vi "Main.vi"() -> ()   [LabVIEW 2016]
uses:
  State.ctl
  <vilib>/DAQmx/write.llb/DAQmx Write (Digital Bool 1Line 1Point).vi
  <vilib>/DAQmx/read.llb/DAQmx Read (Digital Bool 1Line 1Point).vi
  <vilib>/DAQmx/create/channels.llb/DAQmx Create Channel (DI-Digital Input).vi
  <vilib>/DAQmx/create/channels.llb/DAQmx Create Channel (DO-Digital Output).vi
  <vilib>/DAQmx/miscellaneous.llb/DAQmx Fill In Error Info.vi
panel:
  out "Path":path
  out "Pegs Left":dbl
  out "Rings Left":dbl
  in  "Reject Control":bool
  in  "Hopper Control":bool
  in  "Sort  Control":bool
  out "Hopper  Actuator":bool
  out "Reject Solenoid":bool
  out "Sort Solenoid":bool
  in  "Feeder Control":bool
  out "No. Rings Rej":dbl
  out "No. Pegs Rej":dbl
  in  "Belt Control":bool
  out "Rings":dbl
  out "Pegs":dbl
  out "No. Rejected":dbl
  out "No.  Assembled":dbl
  out "Ring Queue":dbl
  out "Reject Solenoid Return":bool
  out "Reject Area Detect":bool
  out "Sensing Area Detect":bool
  out "Sensing Ring Detect":bool
  out "Sensing Peg Detect":bool
  out "Hopper Full":bool
  out "Sort Solenoid Return":bool
  out "Feeder Light":bool
  out "Belt Light":bool
  out "Sort Metal Peg Detect":bool
  out "State":T1
  out "Sorting Area Detect":bool
  out "Off Light":bool
  out "Pause light":bool
  out "On light":bool
  in  "Reset Button":bool
  in  "Abort & Exit Button":bool
  in  "Stop Button":bool
  in  "Pause Button":bool
  in  "Play Button":bool
  out "Peg Flag":bool
  out "Rejection Control":i8
  out "Assembly Flag":bool
  out "Program Control":bool
  # "System Data"
  # "Sensors Panel"
  # "STATUS"
  # "STOP"
  # "READY"
  # "GO!"
  # "ICT3 Controller \nMSE 310 Course Project\nNavjot Singh - 301277656\nNeeraj Bansal - 301323495\nElvis Eshikena - 301302117\nSep - Nov 2018"
  # "Actuators Panel"
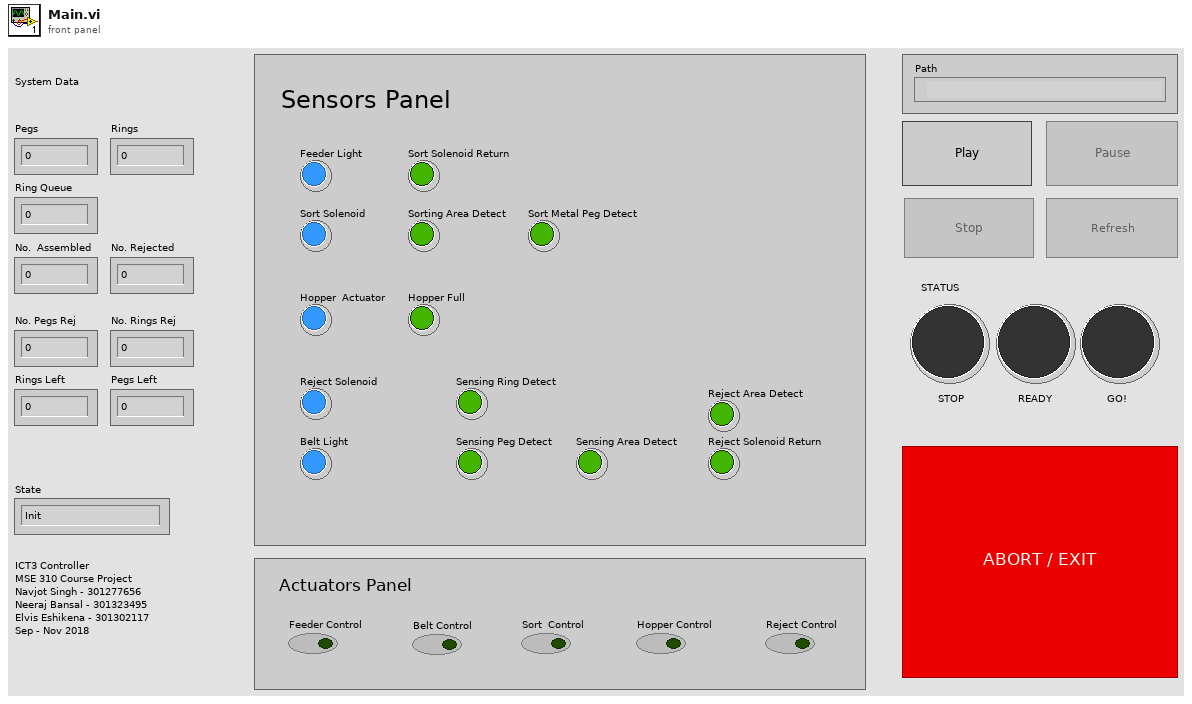
[diagram p1: front panel]
types:
  T1 = typedef "State.ctl" = enum16{"Init", "Idle", "Play", "Pause", "Reset", "Stop", "Stop Program"}
  T2 = enum8{"Enabled", "Disabled", "Disabled and Grayed Out"}
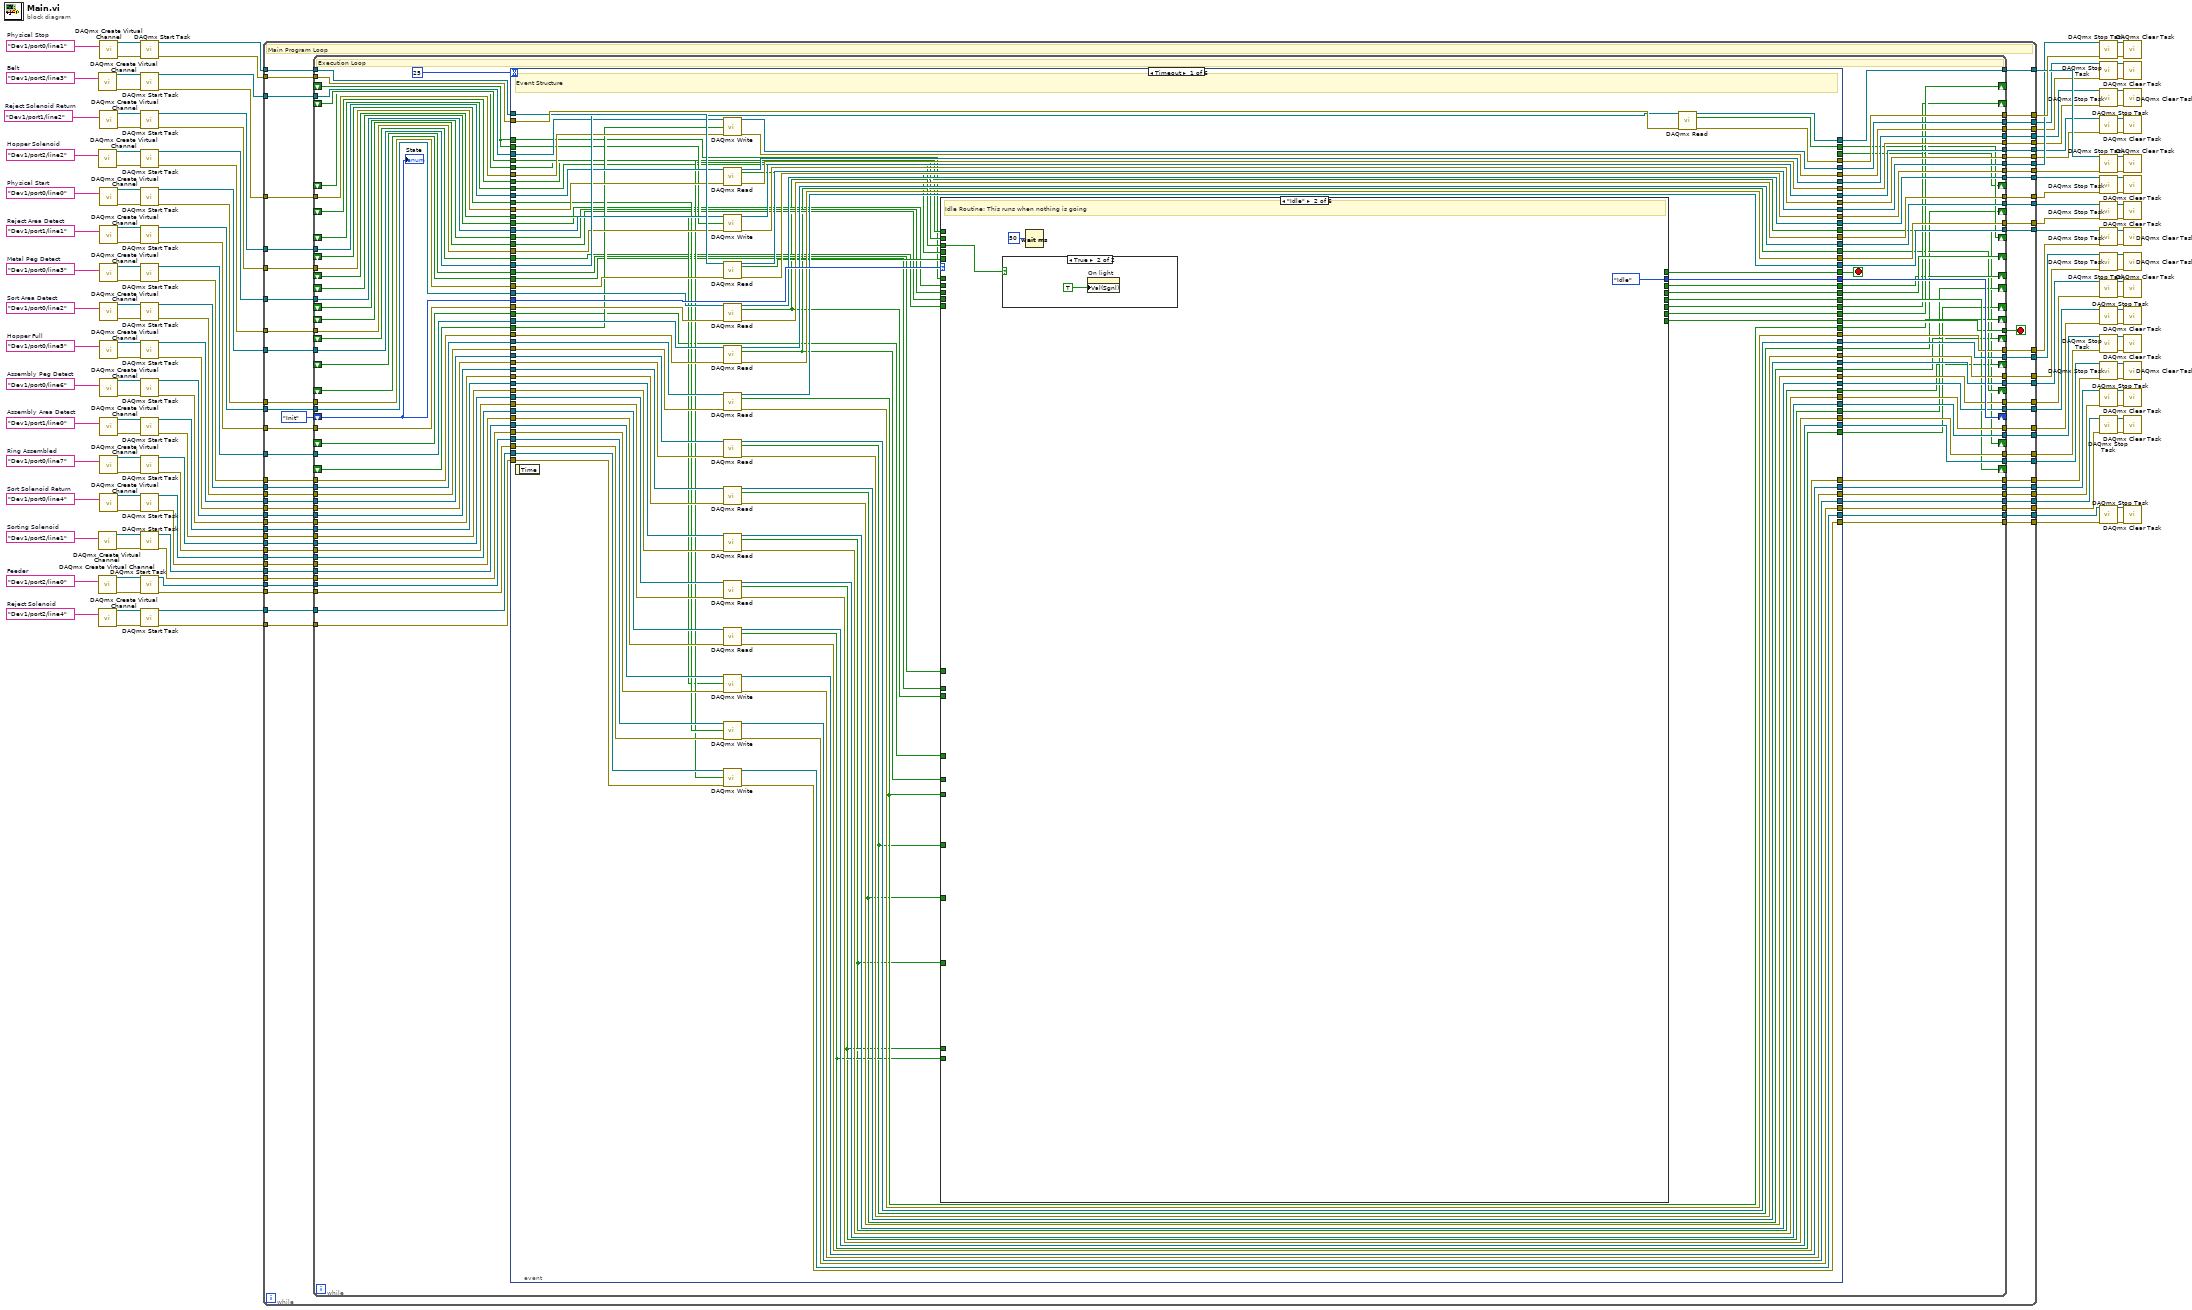
[diagram p0: block diagram]
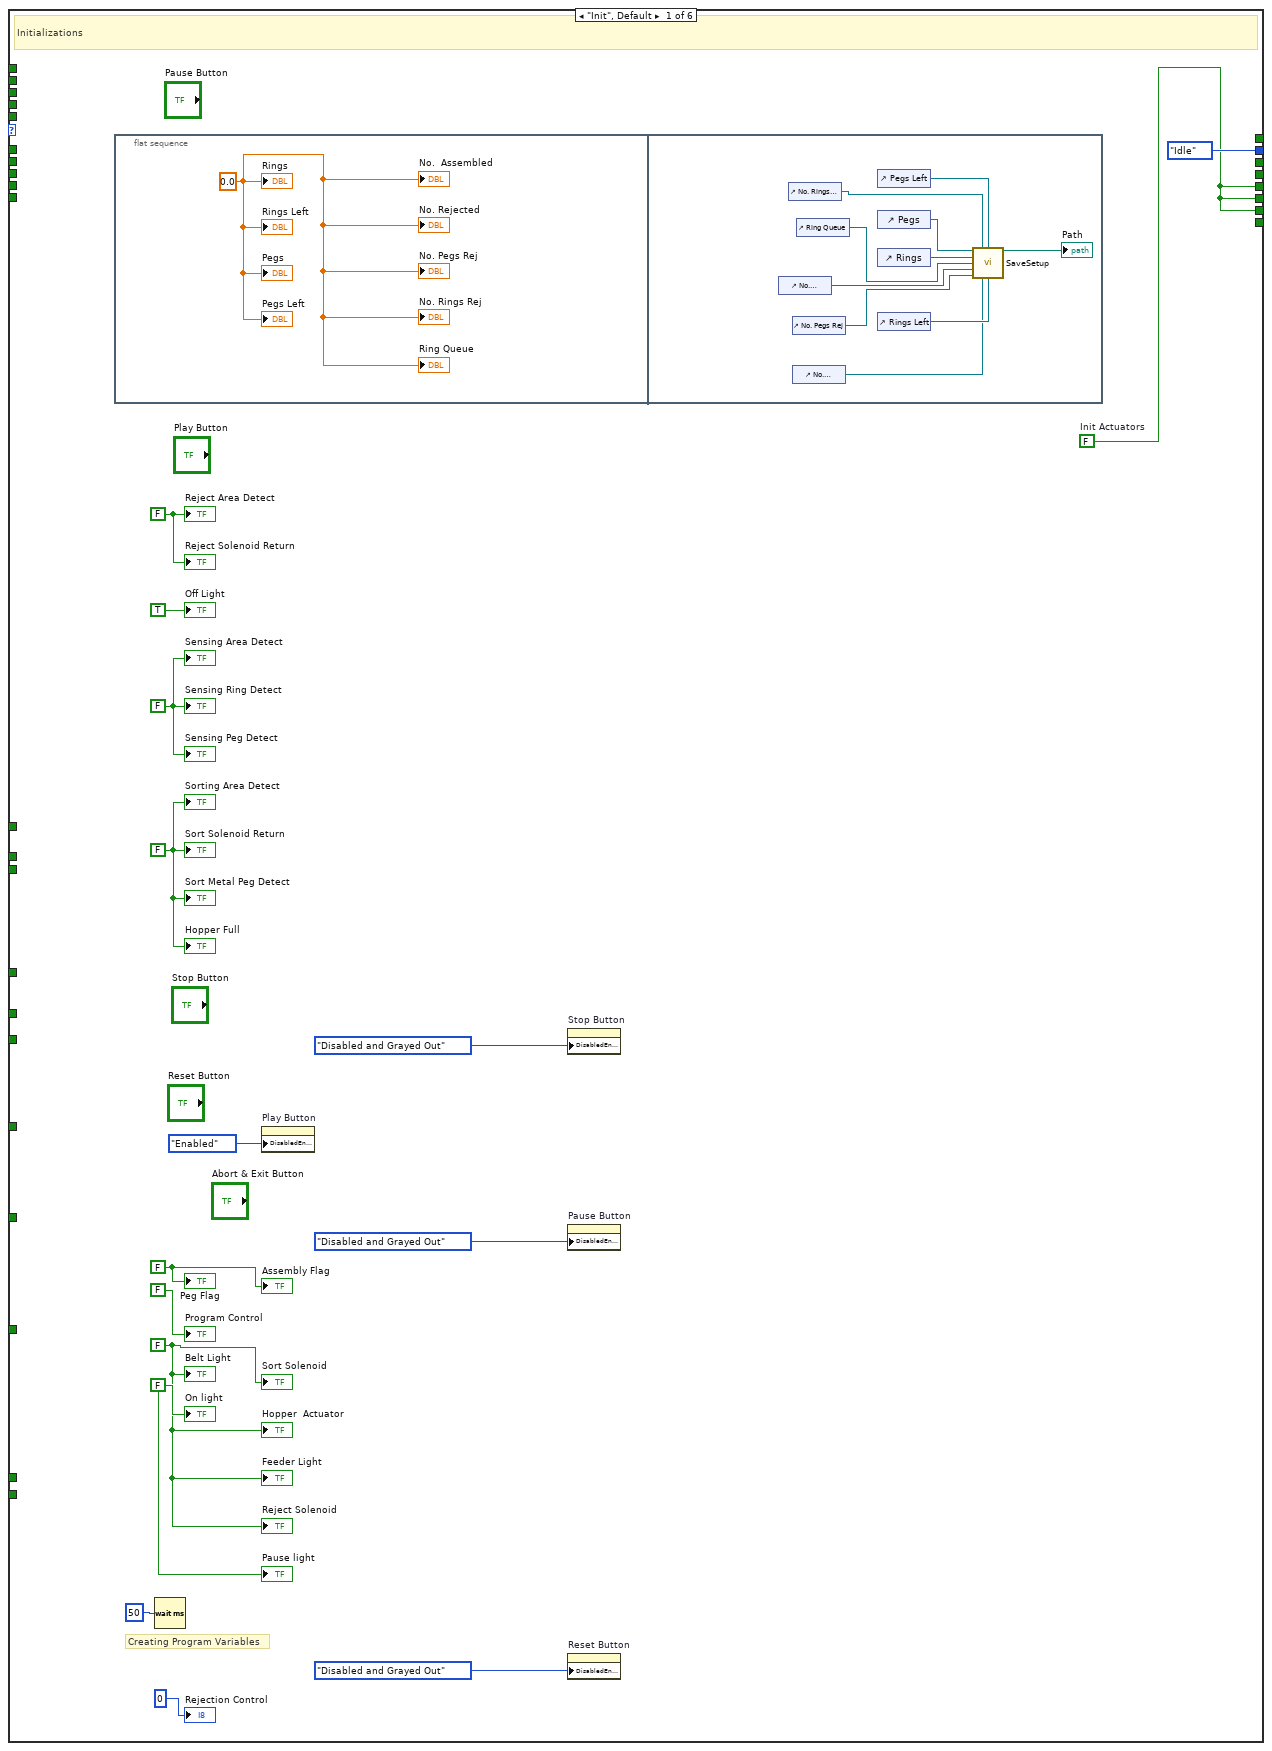
[diagram p2: hidden frame]
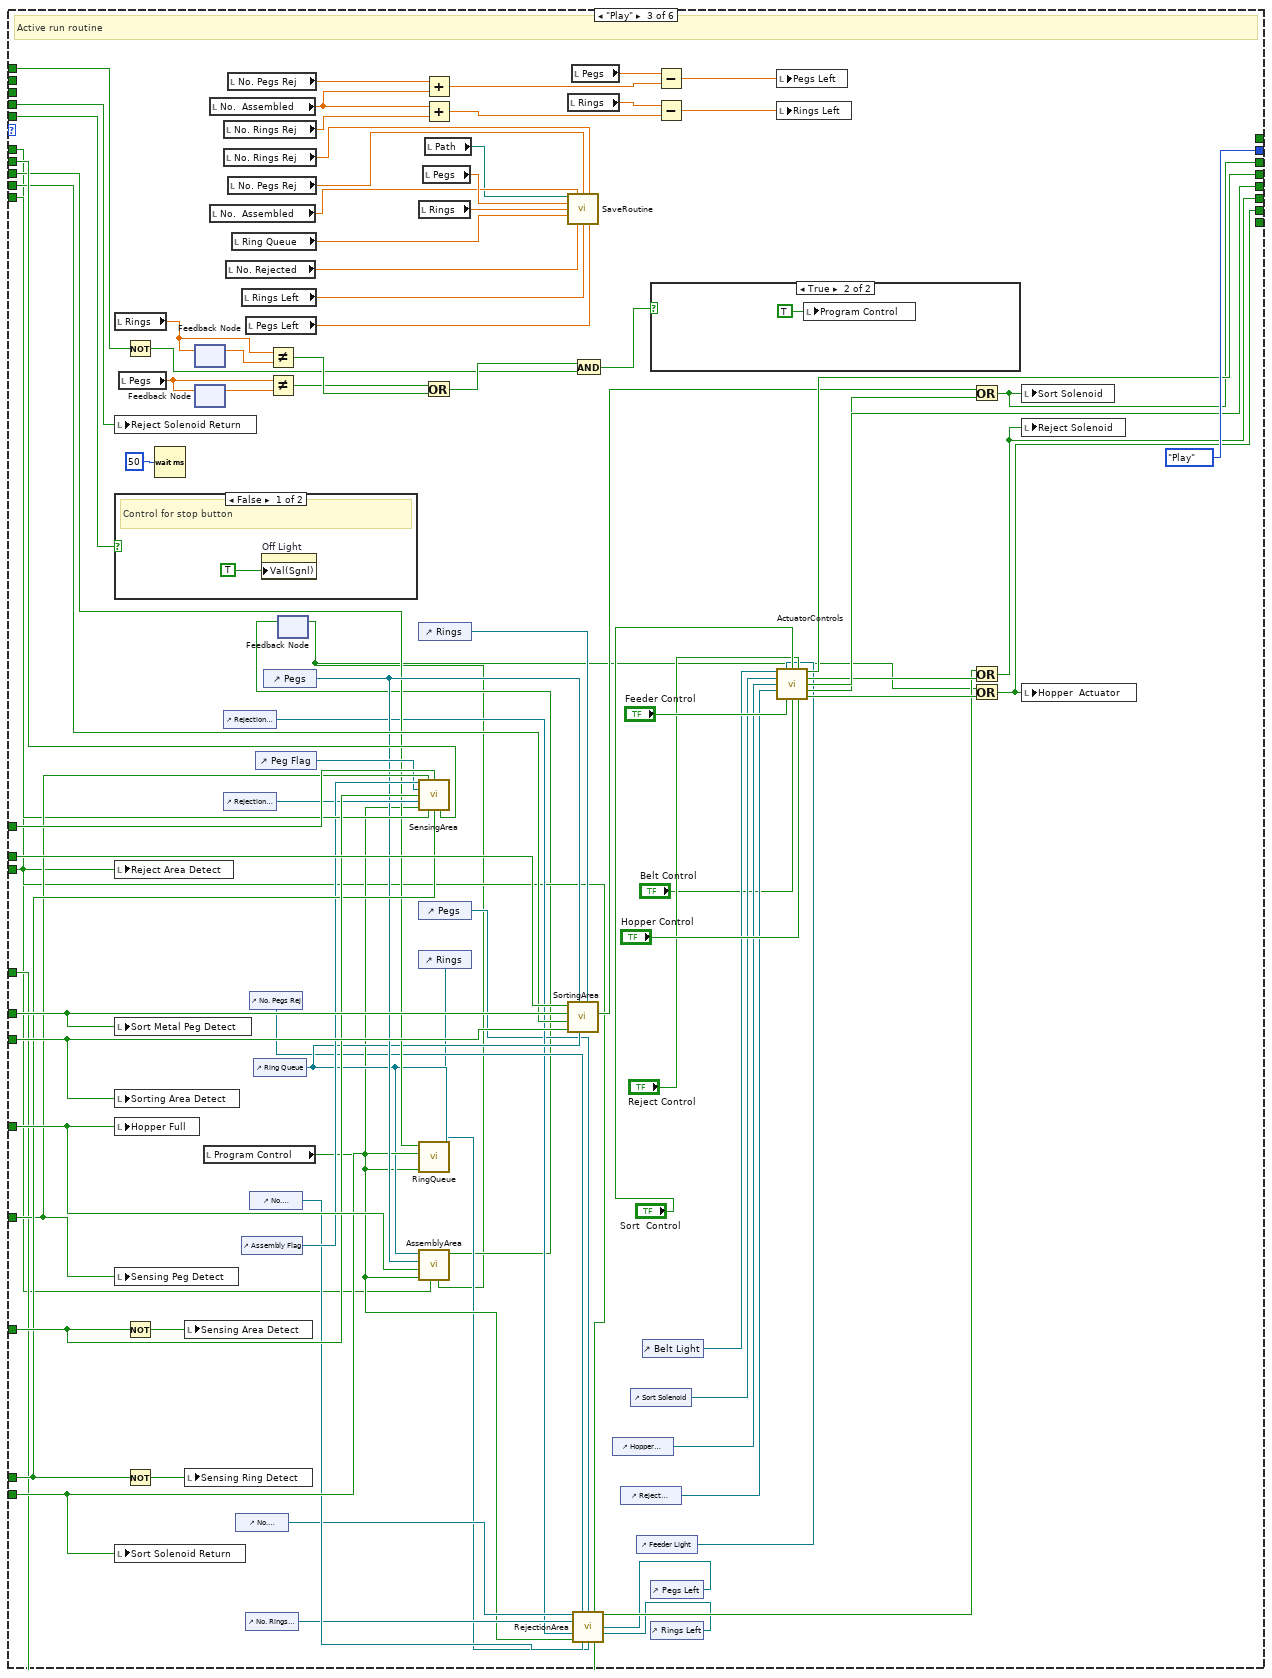
[diagram p4: hidden frame]
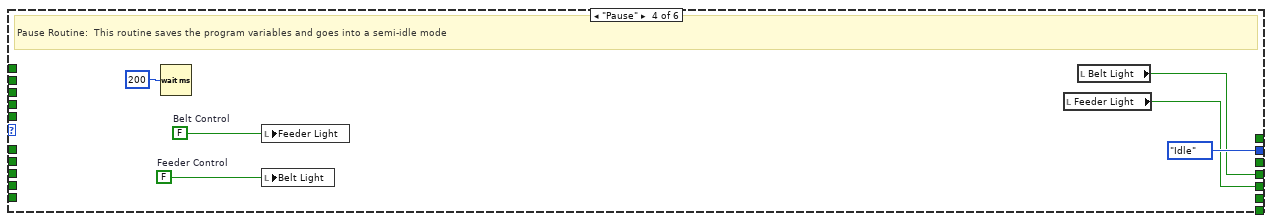
[diagram p7: hidden frame]
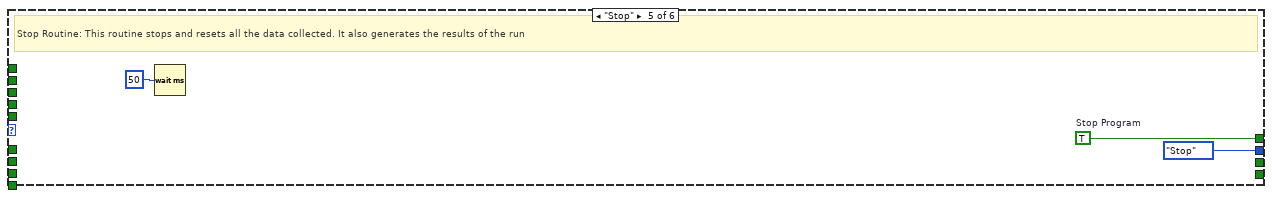
[diagram p8: hidden frame]
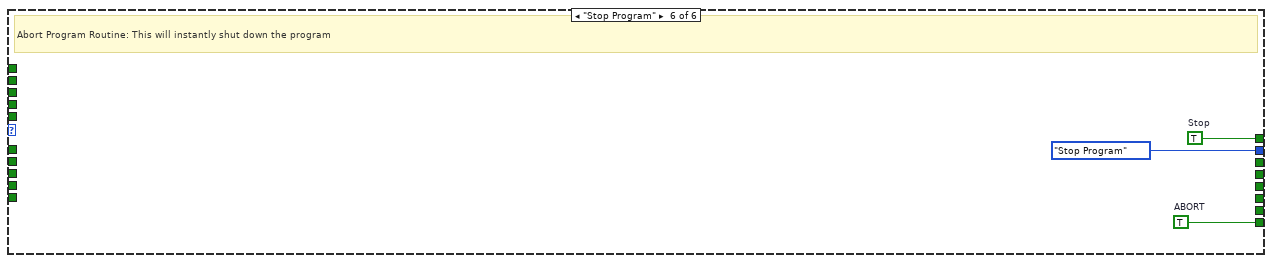
[diagram p9: hidden frame]
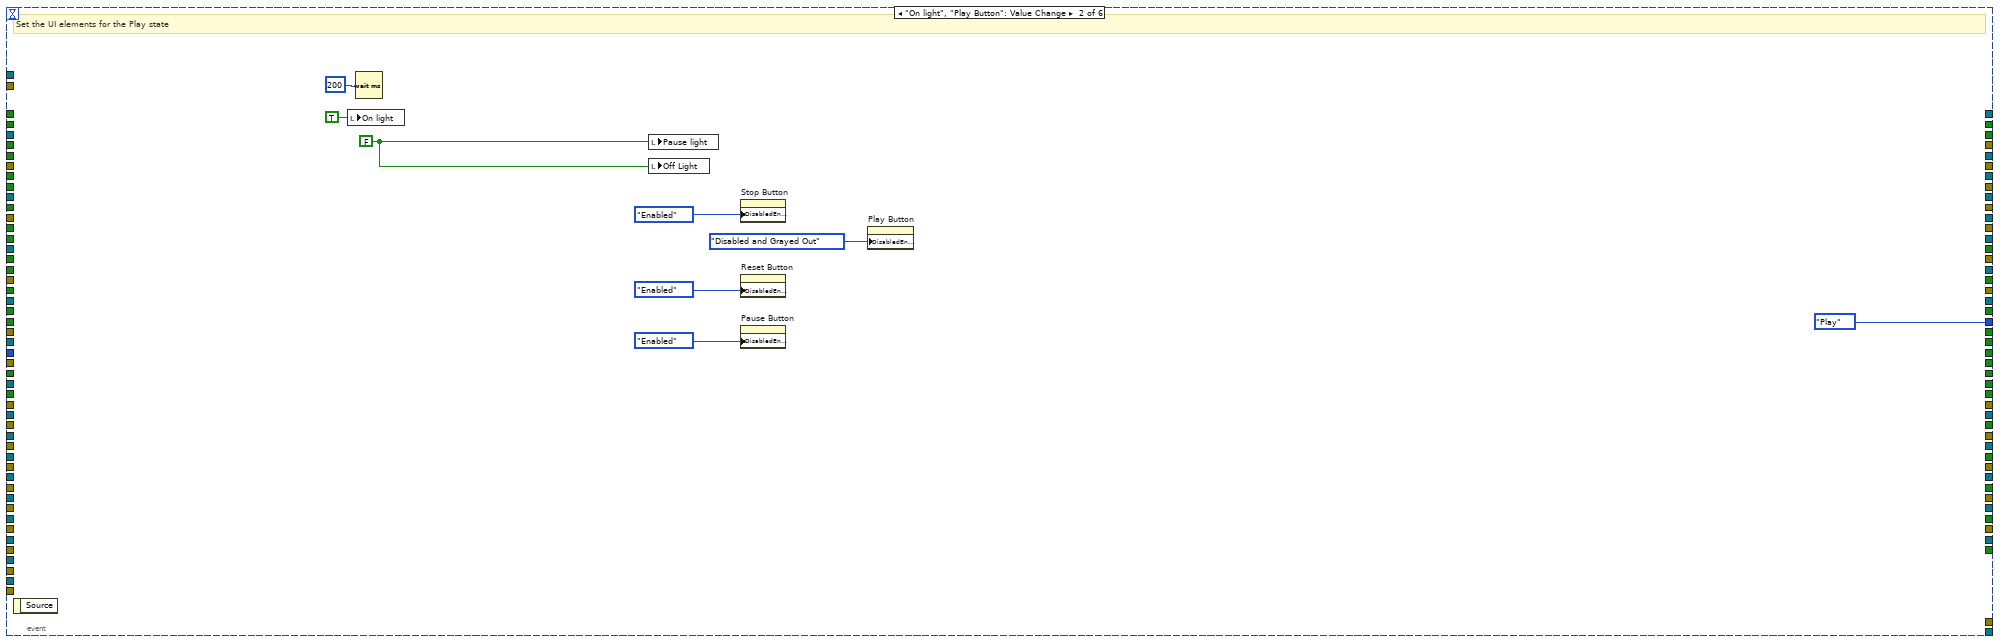
[diagram p10: hidden frame]
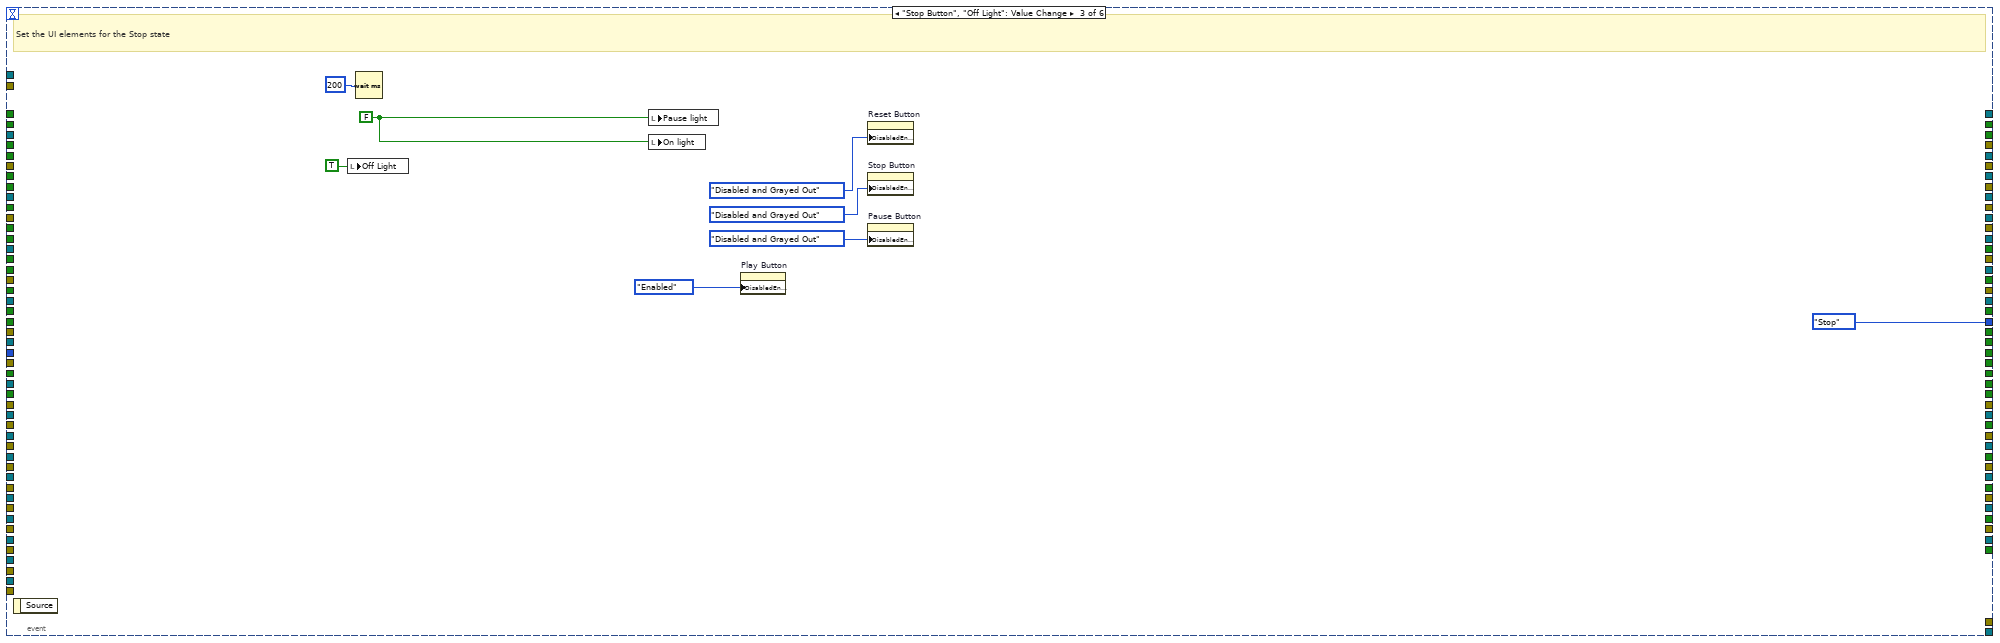
[diagram p11: hidden frame]
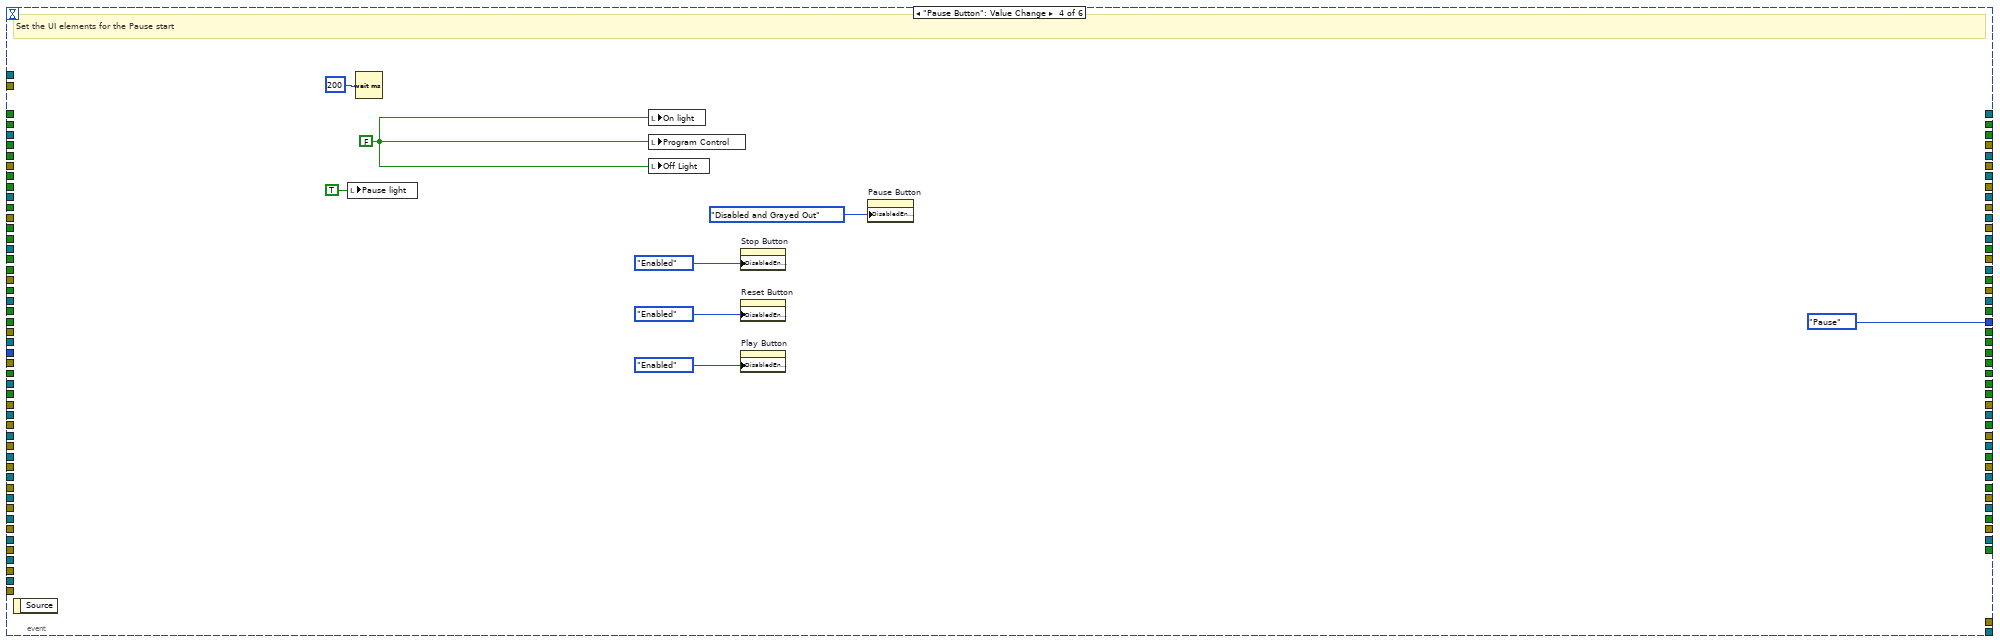
[diagram p12: hidden frame]
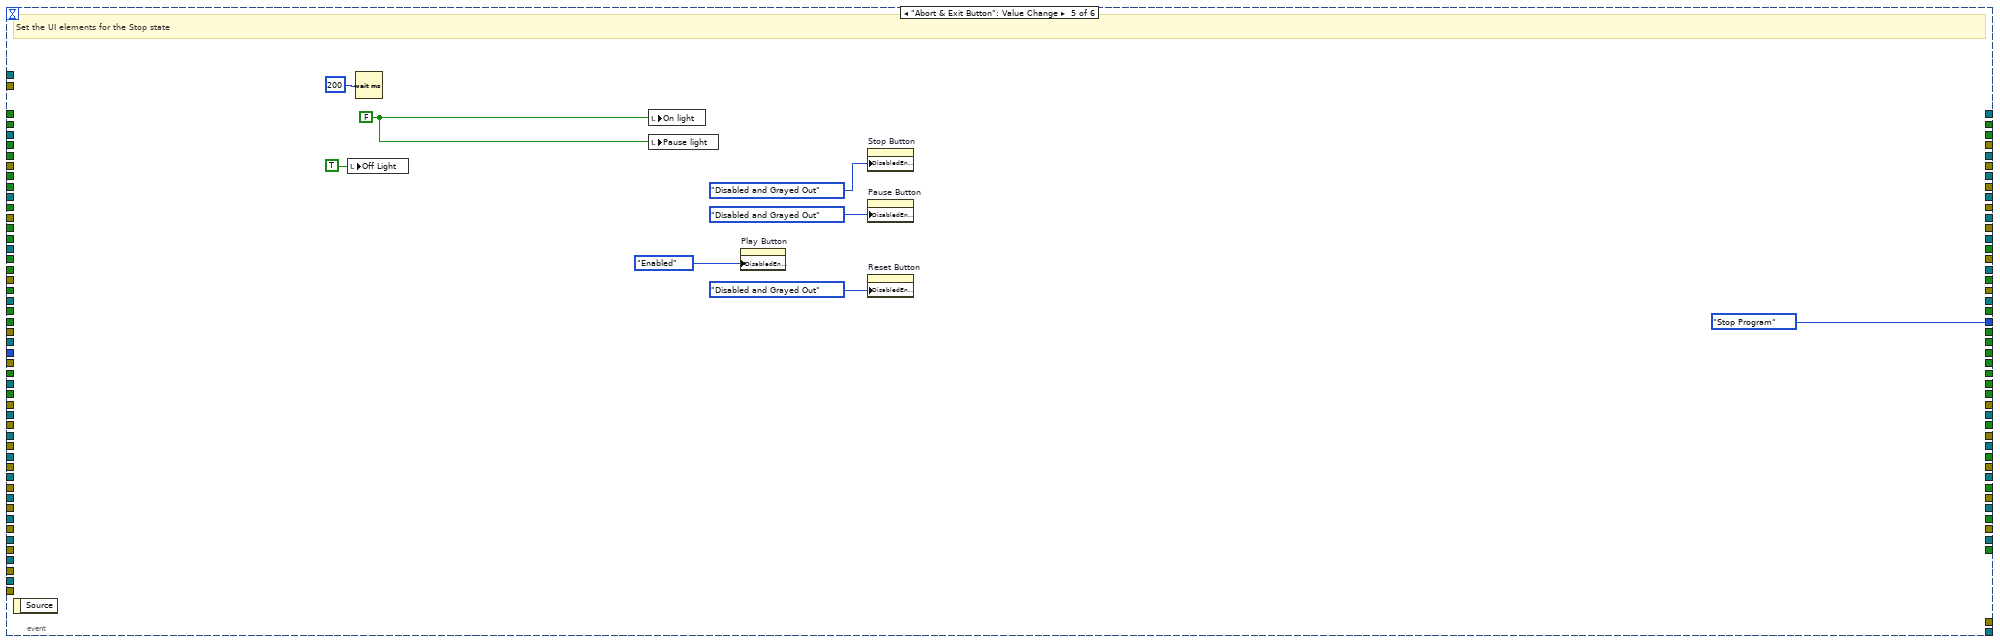
[diagram p13: hidden frame]
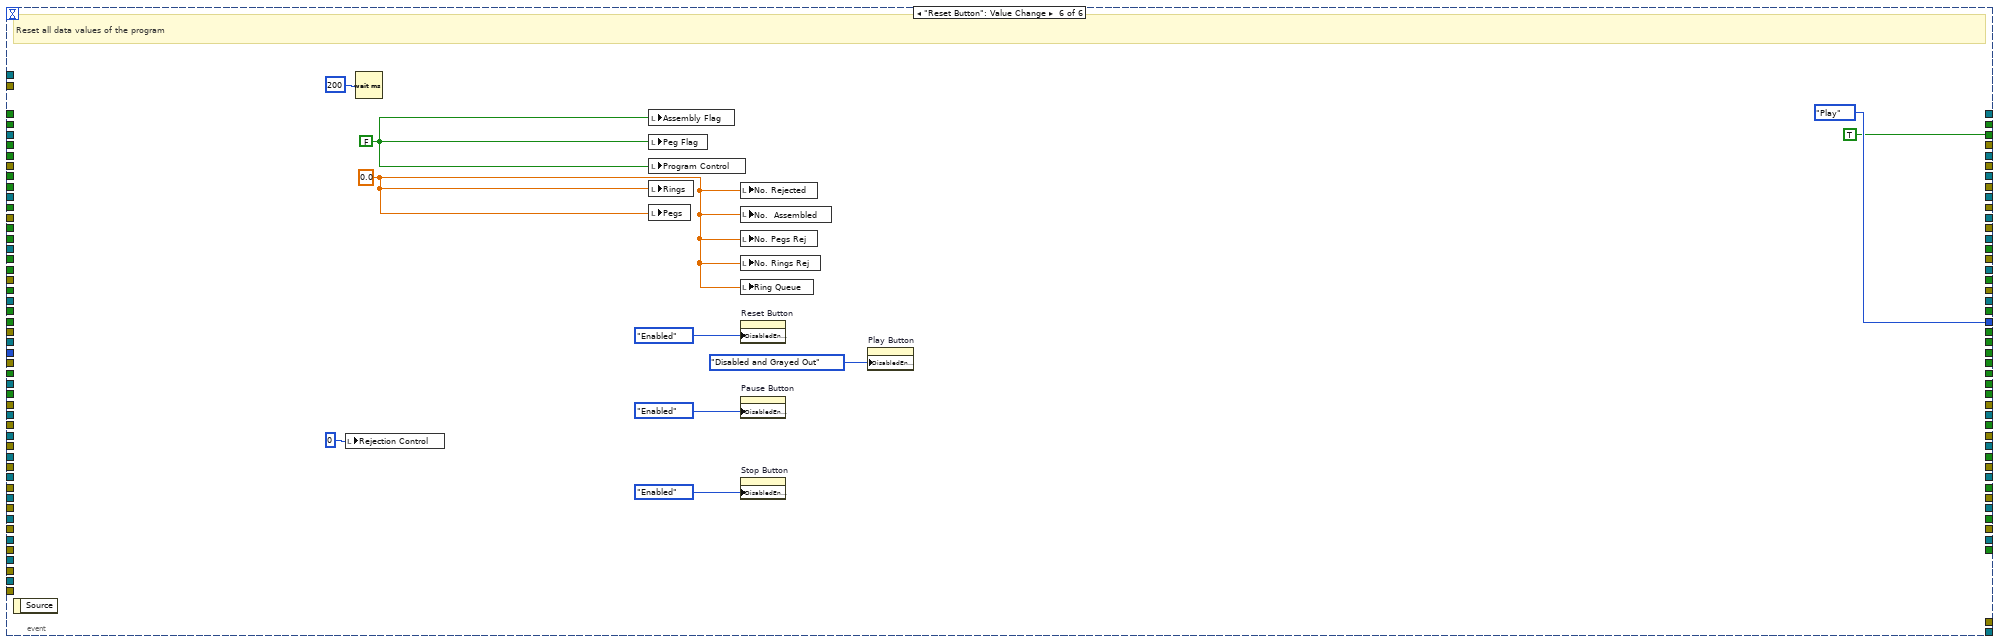
[diagram p14: hidden frame]
diagram:
  w1 = tag "Dev1/port2/line4"  # Reject Solenoid
  w72 = tag "Dev1/port2/line3"  # Belt
  w73 = tag "Dev1/port2/line2"  # Hopper Solenoid
  w74 = tag "Dev1/port2/line1"  # Sorting Solenoid
  w75 = tag "Dev1/port2/line0"  # Feeder
  w76 = tag "Dev1/port1/line2"  # Reject Solenoid Return
  w77 = tag "Dev1/port1/line1"  # Reject Area Detect
  w78 = tag "Dev1/port1/line0"  # Assembly Area Detect
  w79 = tag "Dev1/port0/line7"  # Ring Assembled
  w80 = tag "Dev1/port0/line6"  # Assembly Peg Detect
  w81 = tag "Dev1/port0/line5"  # Hopper Full
  w108 = tag "Dev1/port0/line4"  # Sort Solenoid Return
  w109 = tag "Dev1/port0/line3"  # Metal Peg Detect
  w110 = tag "Dev1/port0/line2"  # Sort Area Detect
  w111 = tag "Dev1/port0/line1"  # Physical Stop
  w112 = tag "Dev1/port0/line0"  # Physical Start
  n1 = call-poly <vilib>:"DAQmx Create Virtual Channel.vi"("lines"=w72) -> ("task out"=w83:refnum<k21>, "error out"=w82:errorcluster)  [unwired: 13 in]
  n2 = call-poly <vilib>:"DAQmx Create Virtual Channel.vi"("lines"=w73) -> ("task out"=w84:refnum<k21>, "error out"=w85:errorcluster)  [unwired: 13 in]
  n3 = call-poly <vilib>:"DAQmx Create Virtual Channel.vi"("lines"=w74) -> ("task out"=w86:refnum<k21>, "error out"=w87:errorcluster)  [unwired: 13 in]
  n4 = call-poly <vilib>:"DAQmx Create Virtual Channel.vi"("lines"=w75) -> ("task out"=w88:refnum<k21>, "error out"=w89:errorcluster)  [unwired: 13 in]
  n5 = call-poly <vilib>:"DAQmx Create Virtual Channel.vi"("lines"=w1) -> ("task out"=w71:refnum<k21>, "error out"=w70:errorcluster)  [unwired: 13 in]
  n6 = call-poly <vilib>:"DAQmx Create Virtual Channel.vi"("lines"=w111) -> ("task out"=w137:refnum<k21>, "error out"=w138:errorcluster)  [unwired: 13 in]
  n7 = call-poly <vilib>:"DAQmx Create Virtual Channel.vi"("lines"=w76) -> ("task out"=w90:refnum<k21>, "error out"=w91:errorcluster)  [unwired: 13 in]
  n8 = call-poly <vilib>:"DAQmx Create Virtual Channel.vi"("lines"=w112) -> ("task out"=w141:refnum<k21>, "error out"=w142:errorcluster)  [unwired: 13 in]
  n9 = call-poly <vilib>:"DAQmx Create Virtual Channel.vi"("lines"=w77) -> ("task out"=w92:refnum<k21>, "error out"=w93:errorcluster)  [unwired: 13 in]
  n10 = call-poly <vilib>:"DAQmx Create Virtual Channel.vi"("lines"=w109) -> ("task out"=w129:refnum<k21>, "error out"=w130:errorcluster)  [unwired: 13 in]
  n11 = call-poly <vilib>:"DAQmx Create Virtual Channel.vi"("lines"=w110) -> ("task out"=w133:refnum<k21>, "error out"=w134:errorcluster)  [unwired: 13 in]
  n12 = call-poly <vilib>:"DAQmx Create Virtual Channel.vi"("lines"=w81) -> ("task out"=w100:refnum<k21>, "error out"=w101:errorcluster)  [unwired: 13 in]
  n13 = call-poly <vilib>:"DAQmx Create Virtual Channel.vi"("lines"=w80) -> ("task out"=w98:refnum<k21>, "error out"=w99:errorcluster)  [unwired: 13 in]
  n14 = call-poly <vilib>:"DAQmx Create Virtual Channel.vi"("lines"=w78) -> ("task out"=w94:refnum<k21>, "error out"=w95:errorcluster)  [unwired: 13 in]
  n15 = call-poly <vilib>:"DAQmx Create Virtual Channel.vi"("lines"=w79) -> ("task out"=w96:refnum<k21>, "error out"=w97:errorcluster)  [unwired: 13 in]
  n16 = call-poly <vilib>:"DAQmx Create Virtual Channel.vi"("lines"=w108) -> ("task out"=w115:refnum<k21>, "error out"=w116:errorcluster)  [unwired: 13 in]
  n17 = call <vilib>:"DAQmx Start Task.vi"("task/channels in"=w137, "error in"=w138) -> ("task out"=w105:refnum<k21>, "error out"=w128:errorcluster)  [unwired: 12 in]
  n18 = call <vilib>:"DAQmx Start Task.vi"("task/channels in"=w83, "error in"=w82) -> ("task out"=w51:refnum<k21>, "error out"=w50:errorcluster)  [unwired: 12 in]
  n19 = call <vilib>:"DAQmx Start Task.vi"("task/channels in"=w90, "error in"=w91) -> ("task out"=w59:refnum<k21>, "error out"=w58:errorcluster)  [unwired: 12 in]
  n20 = call <vilib>:"DAQmx Start Task.vi"("task/channels in"=w84, "error in"=w85) -> ("task out"=w53:refnum<k21>, "error out"=w52:errorcluster)  [unwired: 12 in]
  n21 = call <vilib>:"DAQmx Start Task.vi"("task/channels in"=w141, "error in"=w142) -> ("task out"=w104:refnum<k21>, "error out"=w118:errorcluster)  [unwired: 12 in]
  n22 = call <vilib>:"DAQmx Start Task.vi"("task/channels in"=w92, "error in"=w93) -> ("task out"=w61:refnum<k21>, "error out"=w60:errorcluster)  [unwired: 12 in]
  n23 = call <vilib>:"DAQmx Start Task.vi"("task/channels in"=w129, "error in"=w130) -> ("task out"=w122:refnum<k21>, "error out"=w121:errorcluster)  [unwired: 12 in]
  n24 = call <vilib>:"DAQmx Start Task.vi"("task/channels in"=w133, "error in"=w134) -> ("task out"=w126:refnum<k21>, "error out"=w125:errorcluster)  [unwired: 12 in]
  n25 = call <vilib>:"DAQmx Start Task.vi"("task/channels in"=w100, "error in"=w101) -> ("task out"=w69:refnum<k21>, "error out"=w68:errorcluster)  [unwired: 12 in]
  n26 = call <vilib>:"DAQmx Start Task.vi"("task/channels in"=w98, "error in"=w99) -> ("task out"=w67:refnum<k21>, "error out"=w66:errorcluster)  [unwired: 12 in]
  n27 = call <vilib>:"DAQmx Start Task.vi"("task/channels in"=w94, "error in"=w95) -> ("task out"=w63:refnum<k21>, "error out"=w62:errorcluster)  [unwired: 12 in]
  n28 = call <vilib>:"DAQmx Start Task.vi"("task/channels in"=w96, "error in"=w97) -> ("task out"=w65:refnum<k21>, "error out"=w64:errorcluster)  [unwired: 12 in]
  n29 = call <vilib>:"DAQmx Start Task.vi"("task/channels in"=w115, "error in"=w116) -> ("task out"=w114:refnum<k21>, "error out"=w113:errorcluster)  [unwired: 12 in]
  n30 = call <vilib>:"DAQmx Start Task.vi"("task/channels in"=w86, "error in"=w87) -> ("task out"=w55:refnum<k21>, "error out"=w54:errorcluster)  [unwired: 12 in]
  n31 = call <vilib>:"DAQmx Start Task.vi"("task/channels in"=w88, "error in"=w89) -> ("task out"=w57:refnum<k21>, "error out"=w56:errorcluster)  [unwired: 12 in]
  n32 = call <vilib>:"DAQmx Start Task.vi"("task/channels in"=w71, "error in"=w70) -> ("task out"=w49:refnum<k21>, "error out"=w48:errorcluster)  [unwired: 12 in]
  n33 = while {
    tunnel: w104 -> [w195]
    tunnel: [w194] -> w103
    tunnel: w118 -> [w200]
    tunnel: [w199] -> w117
    tunnel: w105 -> [w196]
    tunnel: [w193] -> w102
    tunnel: w128 -> [w210]
    tunnel: [w209] -> w127
    tunnel: w48 -> [w171]
    tunnel: [w147] -> w2
    tunnel: w49 -> [w172]
    tunnel: [w148] -> w3
    tunnel: w50 -> [w173]
    tunnel: [w149] -> w4
    tunnel: w53 -> [w176]
    tunnel: [w152] -> w7
    tunnel: w51 -> [w174]
    tunnel: [w150] -> w5
    tunnel: w52 -> [w175]
    tunnel: [w151] -> w6
    tunnel: w55 -> [w178]
    tunnel: [w154] -> w9
    tunnel: w54 -> [w177]
    tunnel: [w153] -> w8
    tunnel: w57 -> [w180]
    tunnel: [w156] -> w11
    tunnel: w56 -> [w179]
    tunnel: [w155] -> w10
    tunnel: w58 -> [w181]
    tunnel: [w157] -> w12
    tunnel: w59 -> [w182]
    tunnel: [w158] -> w13
    tunnel: w60 -> [w183]
    tunnel: [w159] -> w14
    tunnel: w61 -> [w184]
    tunnel: [w160] -> w15
    tunnel: w126 -> [w208]
    tunnel: [w206] -> w124
    tunnel: w125 -> [w207]
    tunnel: [w205] -> w123
    tunnel: w122 -> [w204]
    tunnel: [w201] -> w119
    tunnel: w121 -> [w203]
    tunnel: [w202] -> w120
    tunnel: w114 -> [w198]
    tunnel: [w170] -> w47
    tunnel: w113 -> [w197]
    tunnel: [w169] -> w46
    tunnel: w69 -> [w192]
    tunnel: [w168] -> w23
    tunnel: w68 -> [w191]
    tunnel: [w167] -> w22
    tunnel: w67 -> [w190]
    tunnel: [w166] -> w21
    tunnel: w66 -> [w189]
    tunnel: [w165] -> w20
    tunnel: w65 -> [w188]
    tunnel: [w164] -> w19
    tunnel: w62 -> [w185]
    tunnel: [w161] -> w16
    tunnel: w64 -> [w187]
    tunnel: [w163] -> w18
    tunnel: w63 -> [w186]
    tunnel: [w162] -> w17
    stop <- w145 stop-if-true
    # "Main Program Loop"
    n34 = while {
      tunnel: w200 -> [w307]
      tunnel: [w306] -> w199
      tunnel: w210 -> [w309]
      tunnel: [w308] -> w209
      tunnel: w208 -> [w302]
      tunnel: [w300] -> w206
      tunnel: w207 -> [w301]
      tunnel: [w299] -> w205
      tunnel: w204 -> [w298]
      tunnel: [w295] -> w201
      tunnel: w203 -> [w297]
      tunnel: [w296] -> w202
      tunnel: w198 -> [w290]
      tunnel: w197 -> [w289]
      shift-right: [w304] -> _
      shift-left: State."Init" ("State") -> [w214]
      tunnel: w196 -> [w294]
      tunnel: w195 -> [w293]
      tunnel: [w292] -> w194
      tunnel: [w291] -> w193
      tunnel: w192 -> [w288]
      tunnel: w191 -> [w287]
      tunnel: w190 -> [w286]
      tunnel: w189 -> [w285]
      tunnel: w188 -> [w284]
      tunnel: w187 -> [w283]
      tunnel: w186 -> [w282]
      tunnel: w185 -> [w281]
      tunnel: w184 -> [w280]
      tunnel: w183 -> [w279]
      tunnel: w182 -> [w278]
      tunnel: w181 -> [w277]
      tunnel: w180 -> [w276]
      tunnel: w179 -> [w275]
      tunnel: w178 -> [w274]
      tunnel: w177 -> [w273]
      tunnel: w176 -> [w272]
      tunnel: w175 -> [w271]
      tunnel: w174 -> [w270]
      tunnel: w173 -> [w269]
      tunnel: w172 -> [w268]
      tunnel: w171 -> [w267]
      tunnel: [w266] -> w170
      tunnel: [w265] -> w169
      tunnel: [w264] -> w168
      tunnel: [w263] -> w167
      tunnel: [w262] -> w166
      tunnel: [w261] -> w165
      tunnel: [w260] -> w164
      tunnel: [w259] -> w163
      tunnel: [w258] -> w162
      tunnel: [w257] -> w161
      tunnel: [w256] -> w160
      tunnel: [w255] -> w159
      tunnel: [w254] -> w158
      tunnel: [w253] -> w157
      tunnel: [w252] -> w156
      tunnel: [w251] -> w155
      tunnel: [w250] -> w154
      tunnel: [w249] -> w153
      tunnel: [w248] -> w152
      tunnel: [w247] -> w151
      tunnel: [w246] -> w150
      tunnel: [w245] -> w149
      tunnel: [w244] -> w148
      tunnel: [w243] -> w147
      shift-right: [w242] -> _
      shift-left: _ -> [w241]
      shift-right: [w240] -> _
      shift-left: _ -> [w239]
      shift-right: [w238] -> _
      shift-left: _ -> [w211]
      shift-right: [w237] -> _
      shift-left: _ -> [w236]
      shift-right: [w235] -> _
      shift-left: _ -> [w234]
      tunnel: [w233] -> w145
      shift-right: [w232] -> _
      shift-left: _ -> [w231]
      shift-right: [w230] -> _
      shift-left: _ -> [w229]
      shift-right: [w228] -> _
      shift-left: _ -> [w227]
      shift-right: [w226] -> _
      shift-left: _ -> [w225]
      shift-right: [w224] -> _
      shift-left: _ -> [w223]
      shift-right: [w222] -> _
      shift-left: _ -> [w221]
      shift-right: [w220] -> _
      shift-left: _ -> [w219]
      shift-right: [w218] -> _
      shift-left: _ -> [w217]
      shift-right: [w216] -> _
      shift-left: _ -> [w215]
      shift-right: [w213] -> _
      shift-left: _ -> [w212]
      stop <- w303 stop-if-true
      # "Execution Loop"
      n35 = event shown="[0] Timeout" {
        selector: _ -> [_ _ _ _ _ _]
        dyn-events: _ -> [_ _ _ _ _ _]
        timeout: 25 -> [_ _ _ _ _ _]
        tunnel: w309 -> [w405 _ _ _ _ _]
        tunnel: [w402 _ _ _ _ _] -> w308
        tunnel: [w404 _ _ _ _ _] -> w292
        tunnel: w307 -> [w406 _ _ _ _ _]
        tunnel: [w403 _ _ _ _ _] -> w306
        tunnel: w214 -> [w409 _ _ _ _ _]
        tunnel: [w408 State."Play" ("State") State."Stop" ("State") State."Pause" ("State") State."Stop Program" ("State") State."Play" ("State")] -> w304
        tunnel: [w407 _ _ _ _ _] -> w303
        tunnel: w302 -> [w401 _ _ _ _ _]
        tunnel: w301 -> [w400 _ _ _ _ _]
        tunnel: [w398 _ _ _ _ _] -> w300
        tunnel: [w399 _ _ _ _ _] -> w299
        tunnel: w298 -> [w397 _ _ _ _ _]
        tunnel: w297 -> [w396 _ _ _ _ _]
        tunnel: [w395 _ _ _ _ _] -> w296
        tunnel: [w394 _ _ _ _ _] -> w295
        tunnel: w294 -> [w393 _ _ _ _ _]
        tunnel: w293 -> [w392 _ _ _ _ _]
        tunnel: [w391 _ _ _ _ _] -> w291
        tunnel: w290 -> [w390 _ _ _ _ _]
        tunnel: w289 -> [w389 _ _ _ _ _]
        tunnel: w288 -> [w388 _ _ _ _ _]
        tunnel: w287 -> [w387 _ _ _ _ _]
        tunnel: w286 -> [w386 _ _ _ _ _]
        tunnel: w285 -> [w385 _ _ _ _ _]
        tunnel: w284 -> [w384 _ _ _ _ _]
        tunnel: w283 -> [w383 _ _ _ _ _]
        tunnel: w282 -> [w382 _ _ _ _ _]
        tunnel: w281 -> [w381 _ _ _ _ _]
        tunnel: w280 -> [w380 _ _ _ _ _]
        tunnel: w279 -> [w379 _ _ _ _ _]
        tunnel: w278 -> [w378 _ _ _ _ _]
        tunnel: w277 -> [w377 _ _ _ _ _]
        tunnel: w276 -> [w376 _ _ _ _ _]
        tunnel: w275 -> [w375 _ _ _ _ _]
        tunnel: w274 -> [w374 _ _ _ _ _]
        tunnel: w273 -> [w373 _ _ _ _ _]
        tunnel: w272 -> [w372 _ _ _ _ _]
        tunnel: w271 -> [w371 _ _ _ _ _]
        tunnel: w270 -> [w370 _ _ _ _ _]
        tunnel: w269 -> [w369 _ _ _ _ _]
        tunnel: w268 -> [w368 _ _ _ _ _]
        tunnel: w267 -> [w367 _ _ _ _ _]
        tunnel: [w366 _ _ _ _ _] -> w266
        tunnel: [w365 _ _ _ _ _] -> w265
        tunnel: [w364 _ _ _ _ _] -> w264
        tunnel: [w363 _ _ _ _ _] -> w263
        tunnel: [w362 _ _ _ _ _] -> w262
        tunnel: [w361 _ _ _ _ _] -> w261
        tunnel: [w360 _ _ _ _ _] -> w260
        tunnel: [w359 _ _ _ _ _] -> w259
        tunnel: [w358 _ _ _ _ _] -> w258
        tunnel: [w357 _ _ _ _ _] -> w257
        tunnel: [w356 _ _ _ _ _] -> w256
        tunnel: [w355 _ _ _ _ _] -> w255
        tunnel: [w354 _ _ _ _ _] -> w254
        tunnel: [w353 _ _ _ _ _] -> w253
        tunnel: [w352 _ _ _ _ _] -> w252
        tunnel: [w351 _ _ _ _ _] -> w251
        tunnel: [w350 _ _ _ _ _] -> w250
        tunnel: [w349 _ _ _ _ _] -> w249
        tunnel: [w348 _ _ _ _ _] -> w248
        tunnel: [w347 _ _ _ _ _] -> w247
        tunnel: [w346 _ _ _ _ _] -> w246
        tunnel: [w345 _ _ _ _ _] -> w245
        tunnel: [w344 _ _ _ _ _] -> w244
        tunnel: [w343 _ _ _ _ _] -> w243
        tunnel: [w342 _ _ _ _ _] -> w242
        tunnel: w241 -> [w341 _ _ _ _ _]
        tunnel: [w340 _ _ _ _ _] -> w240
        tunnel: w239 -> [w339 _ _ _ _ _]
        tunnel: [w338 _ _ _ _ _] -> w238
        tunnel: w211 -> [w337 _ _ _ _ _]
        tunnel: [w336 _ _ _ _ _] -> w237
        tunnel: w236 -> [w335 _ _ _ _ _]
        tunnel: [w334 _ _ _ _ _] -> w235
        tunnel: w234 -> [w333 _ _ _ _ _]
        tunnel: [w331 _ _ _ _ _] -> w233
        tunnel: [w330 _ _ _ _ _] -> w232
        tunnel: w231 -> [w329 _ _ _ _ _]
        tunnel: [w325 _ _ _ _ _] -> w230
        tunnel: w229 -> [w328 _ _ _ _ _]
        tunnel: [w324 _ _ _ _ _] -> w228
        tunnel: w227 -> [w327 _ _ _ _ _]
        tunnel: [w323 _ _ _ _ _] -> w226
        tunnel: w225 -> [w326 _ _ _ _ _]
        tunnel: [w322 _ _ _ _ _] -> w224
        tunnel: w223 -> [w321 _ _ _ _ _]
        tunnel: [w319 _ _ _ _ _] -> w222
        tunnel: w221 -> [w320 _ _ _ _ _]
        tunnel: [w317 _ _ _ _ _] -> w220
        tunnel: w219 -> [w318 _ _ _ _ _]
        tunnel: [w316 _ _ _ _ _] -> w218
        tunnel: w217 -> [w315 _ _ _ _ _]
        tunnel: [w314 _ _ _ _ _] -> w216
        tunnel: w215 -> [w313 _ _ _ _ _]
        tunnel: [_ _ _ _ _ TRUE] -> w213
        tunnel: w212 -> [w311 _ _ _ _ _]
        tunnel: w211 -> [w310 _ _ _ _ _]
        event Timeout {
          # "Event Structure"
          n36 = event-data() -> ()  [unwired: 1 in, 1 out]
          n37 = call-poly <vilib>:"DAQmx Write.vi"("task/channels in"=w370, "data"=w341, "error in"=w369) -> ("task out"=w346:refnum<k21>, "error out"=w345:errorcluster)  [unwired: 10 in, 1 out]
          n38 = call-poly <vilib>:"DAQmx Read.vi"("task/channels in"=w378, "error in"=w377) -> ("task out"=w354:refnum<k21>, "data"=w312:bool, "error out"=w353:errorcluster)  [unwired: 11 in]
          n39 = call-poly <vilib>:"DAQmx Write.vi"("task/channels in"=w372, "data"=w337, "error in"=w371) -> ("task out"=w348:refnum<k21>, "error out"=w347:errorcluster)  [unwired: 10 in, 1 out]
          n40 = call-poly <vilib>:"DAQmx Read.vi"("task/channels in"=w393, "error in"=w406) -> ("task out"=w391:refnum<k21>, "data"=w332:bool, "error out"=w403:errorcluster)  [unwired: 11 in]
          n41 = call-poly <vilib>:"DAQmx Read.vi"("task/channels in"=w380, "error in"=w379) -> ("task out"=w356:refnum<k21>, "data"=w314:bool, "error out"=w355:errorcluster)  [unwired: 11 in]
          n42 = call-poly <vilib>:"DAQmx Read.vi"("task/channels in"=w397, "error in"=w396) -> ("task out"=w394:refnum<k21>, "data"=w324:bool, "error out"=w395:errorcluster)  [unwired: 11 in]
          n43 = call-poly <vilib>:"DAQmx Read.vi"("task/channels in"=w401, "error in"=w400) -> ("task out"=w398:refnum<k21>, "data"=w325:bool, "error out"=w399:errorcluster)  [unwired: 11 in]
          n44 = call-poly <vilib>:"DAQmx Read.vi"("task/channels in"=w388, "error in"=w387) -> ("task out"=w364:refnum<k21>, "data"=w322:bool, "error out"=w363:errorcluster)  [unwired: 11 in]
          n45 = call-poly <vilib>:"DAQmx Read.vi"("task/channels in"=w386, "error in"=w385) -> ("task out"=w362:refnum<k21>, "data"=w319:bool, "error out"=w361:errorcluster)  [unwired: 11 in]
          n46 = call-poly <vilib>:"DAQmx Read.vi"("task/channels in"=w382, "error in"=w381) -> ("task out"=w358:refnum<k21>, "data"=w316:bool, "error out"=w357:errorcluster)  [unwired: 11 in]
          n47 = call-poly <vilib>:"DAQmx Read.vi"("task/channels in"=w384, "error in"=w383) -> ("task out"=w360:refnum<k21>, "data"=w317:bool, "error out"=w359:errorcluster)  [unwired: 11 in]
          n48 = call-poly <vilib>:"DAQmx Read.vi"("task/channels in"=w390, "error in"=w389) -> ("task out"=w366:refnum<k21>, "data"=w323:bool, "error out"=w365:errorcluster)  [unwired: 11 in]
          n49 = call-poly <vilib>:"DAQmx Write.vi"("task/channels in"=w374, "data"=w329, "error in"=w373) -> ("task out"=w350:refnum<k21>, "error out"=w349:errorcluster)  [unwired: 10 in, 1 out]
          n50 = call-poly <vilib>:"DAQmx Write.vi"("task/channels in"=w376, "data"=w339, "error in"=w375) -> ("task out"=w352:refnum<k21>, "error out"=w351:errorcluster)  [unwired: 10 in, 1 out]
          n51 = call-poly <vilib>:"DAQmx Write.vi"("task/channels in"=w368, "data"=w335, "error in"=w367) -> ("task out"=w344:refnum<k21>, "error out"=w343:errorcluster)  [unwired: 10 in, 1 out]
          n52 = case shown="\"Idle\"" w409 {
            tunnel: [State."Idle" ("State") State."Idle" ("State") State."Play" ("State") State."Idle" ("State") State."Stop" ("State") State."Stop Program" ("State")] -> w408
            tunnel: [_ _ _ _ w538 w542] -> w407
            tunnel: [w416 _ w527 w532 _ _] -> w342
            tunnel: [_ _ w526 w534 _ _] -> w340
            tunnel: [w416 _ w499 _ _ _] -> w338
            tunnel: [w416 _ w498 _ _ _] -> w336
            tunnel: w333 -> [_ w437 _ _ _ _]
            tunnel: w332 -> [_ _ w525 _ _ _]
            tunnel: [_ _ _ _ _ w541] -> w331
            tunnel: w327 -> [_ _ w522 _ _ _]
            tunnel: w326 -> [_ _ w477 _ _ _]
            tunnel: w328 -> [_ _ w491 _ _ _]
            tunnel: [_ _ w497 _ _ _] -> w330
            tunnel: w325 -> [_ _ w524 _ _ _]
            tunnel: w324 -> [_ _ w523 _ _ _]
            tunnel: w323 -> [_ _ w478 _ _ _]
            tunnel: w322 -> [_ _ w521 _ _ _]
            tunnel: w321 -> [_ _ _ _ _ _]
            tunnel: w320 -> [_ _ w513 _ _ _]
            tunnel: w319 -> [_ _ w514 _ _ _]
            tunnel: w318 -> [_ _ w515 _ _ _]
            tunnel: w317 -> [_ _ w516 _ _ _]
            tunnel: w316 -> [_ _ w520 _ _ _]
            tunnel: w315 -> [_ _ w519 _ _ _]
            tunnel: w314 -> [_ _ w469 _ _ _]
            tunnel: w313 -> [_ _ w468 _ _ _]
            tunnel: w312 -> [_ _ w492 _ _ _]
            tunnel: w311 -> [_ _ w482 _ _ _]
            tunnel: w310 -> [_ _ w441 _ _ _]
            frame "Init", Default {
              w416 = FALSE  # Init Actuators
              w421 = FALSE
              w418 = FALSE
              w422 = FALSE ("Sorting Area Detect")
              w415 = FALSE ("Assembly Flag")
              w423 = FALSE
              w417 = FALSE
              # "Creating Program Variables"
              # "Initializations"
              n53 = flat-sequence {
                frame #0 {
                  w426 = 0.0 ("Pegs")
                  "Ring Queue" <- w426
                  "No.  Assembled" <- w426
                  "No. Rejected" <- w426
                  "Pegs" <- w426
                  "Rings" <- w426
                  "No. Pegs Rej" <- w426
                  "No. Rings Rej" <- w426
                  "Rings Left" <- w426
                  "Pegs Left" <- w426
                }
                frame #1 {
                  n54 = control-ref of="No.  Assembled"() -> (w429:refnum<vi>)
                  n55 = control-ref of="No. Rings Rej"() -> (w434:refnum<vi>)
                  n56 = control-ref of="No. Pegs Rej"() -> (w433:refnum<vi>)
                  n57 = control-ref of="No. Rejected"() -> (w430:refnum<vi>)
                  n58 = control-ref of="Ring Queue"() -> (w428:refnum<vi>)
                  n59 = control-ref of="Pegs Left"() -> (w436:refnum<vi>)
                  n60 = control-ref of="Pegs"() -> (w431:refnum<vi>)
                  n61 = control-ref of="Rings"() -> (w432:refnum<vi>)
                  n62 = control-ref of="Rings Left"() -> (w435:refnum<vi>)
                  n63 = call "SaveSetup.vi"("Pegs"=w431, "Rings Rej"=w434, "Pegs Left"=w436, "Rings"=w432, "RingQ"=w428, "No Assem"=w429, "Pegs Rej"=w433, "Total Rej"=w430, "Rings Left"=w435) -> ("Path"=→"Path":path)  [unwired: 6 in]
                }
              }
              n64 = Wait (ms)(milliseconds to wait=u32 50) -> ()  [unwired: 1 out]
              n65 = property on="Play Button" class="Bool"("DisabledEnum"=T2."Enabled" ("Disabled")) -> ()  [unwired: 2 in, 2 out]
              n66 = property on="Stop Button" class="Bool"("DisabledEnum"=T2."Disabled and Grayed Out" ("Disabled")) -> ()  [unwired: 2 in, 2 out]
              n67 = property on="Pause Button" class="Bool"("DisabledEnum"=T2."Disabled and Grayed Out" ("Disabled")) -> ()  [unwired: 2 in, 2 out]
              n68 = property on="Reset Button" class="Bool"("DisabledEnum"=T2."Disabled and Grayed Out" ("Disabled")) -> ()  [unwired: 2 in, 2 out]
              "Pause light" <- w423
              "On light" <- w423
              "Off Light" <- TRUE ("Off Light")
              "Belt Light" <- w417
              "Feeder Light" <- w417
              "Assembly Flag" <- w415
              "Peg Flag" <- w415
              "Sort Metal Peg Detect" <- w422
              "Sorting Area Detect" <- w422
              "Sort Solenoid Return" <- w422
              "Hopper Full" <- w422
              "Sensing Peg Detect" <- w418
              "Sensing Ring Detect" <- w418
              "Sensing Area Detect" <- w418
              "Reject Area Detect" <- w421
              "Reject Solenoid Return" <- w421
              "Rejection Control" <- i8 0 ("Rejection Control")
              "Sort Solenoid" <- w417
              "Reject Solenoid" <- w417
              "Hopper  Actuator" <- w417
              "Program Control" <- FALSE ("Program Control")
            }
            frame "Idle" {
              # "Idle Routine: This runs when nothing is going"
              n69 = case shown="True" w437 {
                frame False {
                }
                frame True {
                  n70 = property on="On light" class="Bool (strict)"("Val(Sgnl)"=TRUE ("Value (Signaling)")) -> ()  [unwired: 2 in, 2 out]
                }
              }
              n71 = Wait (ms)(milliseconds to wait=u32 50 ("millisecond timer value")) -> ()  [unwired: 1 out]
            }
            frame "Play" {
              # "Active run routine"
              n72 = local read "Rings"() -> (w485:dbl)
              n73 = local write "Reject Solenoid Return"(w492) -> ()
              n74 = case shown="False" w525 {
                frame False {
                  # "Control for stop button"
                  n75 = property on="Off Light" class="Bool (strict)"("Val(Sgnl)"=TRUE ("Value (Signaling)")) -> ()  [unwired: 2 in, 2 out]
                }
                frame True {
                }
              }
              n76 = local write "Reject Area Detect"(w469) -> ()
              n77 = local write "Sort Metal Peg Detect"(w523) -> ()
              n78 = local write "Sorting Area Detect"(w524) -> ()
              n79 = local write "Hopper Full"(w521) -> ()
              n80 = local write "Sensing Peg Detect"(w514) -> ()
              n81 = local write "Sort Solenoid Return"(w478) -> ()
              n82 = local read "Pegs"() -> (w487:dbl)
              n83 = Not(x=w482) -> (.not. x?=w479:bool)
              n84 = Not(x=w520) -> (.not. x?=w518:bool)
              n85 = Not(x=w516) -> (.not. x?=w517:bool)
              n86 = Wait (ms)(milliseconds to wait=u32 50 ("millisecond timer value")) -> ()  [unwired: 1 out]
              n87 = local write "Sensing Area Detect"(w518) -> ()
              n88 = local write "Sensing Ring Detect"(w517) -> ()
              n89 = feedback #1() -> (w486:dbl)  [unwired: 1 in]
              n90 = feedback-in #1(w485) -> ()
              n91 = feedback #2() -> (w488:dbl)  [unwired: 1 in]
              n92 = feedback-in #2(w487) -> ()
              n93 = local read "Program Control"() -> (w472:bool)
              n94 = local read "No.  Assembled"() -> (w446:dbl)
              n95 = local read "No.  Assembled"() -> (w455:dbl)
              n96 = local read "No. Rings Rej"() -> (w444:dbl)
              n97 = local read "No. Rings Rej"() -> (w460:dbl)
              n98 = control-ref of="Rejection Control"() -> (w470:refnum<vi>)
              n99 = control-ref of="Rejection Control"() -> (w493:refnum<vi>)
              n100 = local read "No. Rejected"() -> (w456:dbl)
              n101 = local read "No. Pegs Rej"() -> (w445:dbl)
              n102 = local read "No. Pegs Rej"() -> (w459:dbl)
              n103 = local read "Ring Queue"() -> (w454:dbl)
              n104 = control-ref of="No.  Assembled"() -> (w473:refnum<vi>)
              n105 = local read "Rings Left"() -> (w461:dbl)
              n106 = control-ref of="Assembly Flag"() -> (w495:refnum<vi>)
              n107 = local read "Pegs Left"() -> (w462:dbl)
              n108 = control-ref of="No. Rings Rej"() -> (w474:refnum<vi>)
              n109 = control-ref of="No. Pegs Rej"() -> (w471:refnum<vi>)
              n110 = control-ref of="No. Rejected"() -> (w475:refnum<vi>)
              n111 = control-ref of="Ring Queue"() -> (w476:refnum<vi>)
              n112 = control-ref of="Peg Flag"() -> (w494:refnum<vi>)
              n113 = control-ref of="Pegs"() -> (w490:refnum<vi>)
              n114 = Not Equal?(x=w485, y=w486) -> (x != y?=w484:bool)
              n115 = Not Equal?(x=w487, y=w488) -> (x != y?=w483:bool)
              n116 = feedback #3() -> (w442:bool)  [unwired: 1 in]
              n117 = local read "Rings"() -> (w458:dbl)
              n118 = control-ref of="Rings"() -> (w489:refnum<vi>)
              n119 = call "SensingArea.vi"("Assem Flag"=w495, "Metal Curr"=w514, "Sensing Sw Prev"=w519, "Peg Flag"=w494, "Sensing Sw Curr"=w520, "RejectionCntrl"=w493, "Program Control"=w472, "Metal Prev"=w513, "Plastic Current"=w516, "Plastic Previous"=w515) -> ()  [unwired: 6 in]
              n120 = control-ref of="Pegs"() -> (w463:refnum<vi>)
              n121 = control-ref of="Rings"() -> (w464:refnum<vi>)
              n122 = call "RingQueue.vi"("Prev Solenoid Data"=w477, "Curr Solenoid Data"=w478, "Program control"=w472, "RingQueue"=w476) -> ()  [unwired: 7 in]
              n123 = call "AssemblyArea.vi"("Current Hopper Val"=w442, "Prev Hopper Val"=w441, "Program Control"=w472, "Hopper Detect"=w521, "Pegs"=w490, "RingQ"=w476) -> ("Hopper Solenoid"=w443:bool)  [unwired: 5 in]
              n124 = feedback-in #3(w443) -> ()
              n125 = local read "Pegs"() -> (w457:dbl)
              n126 = Add(x=w445, y=w446) -> (x+y=w451:dbl)
              n127 = Add(x=w446, y=w444) -> (x+y=w452:dbl)
              n128 = Or(x=w483, y=w484) -> (x .or. y?=w481:bool)
              n129 = local read "Path"() -> (w453:path)
              n130 = local read "Rings"() -> (w447:dbl)
              n131 = call "SaveRoutine.vi"("Path"=w453, "No. of Assem"=w455, "No. Pegs Rej"=w459, "No. Rings Rej"=w460, "No. Pegs"=w457, "No. of Rings"=w458, "No. RingQ"=w454, "Total Rej"=w456, "Rings Left"=w461, "Pegs Left"=w462) -> ()  [unwired: 6 in]
              n132 = call "SortingArea.vi"("Ring Ref"=w489, "RingQueue Ref"=w476, "Peg Ref"=w490, "Current Area Detect"=w524, "Prev Area Detect"=w491, "Current Metal Detect"=w523, "Prev Metal Detect"=w522) -> ("Sorting Solenoid Out"=w505:bool)  [unwired: 4 in]
              n133 = local read "Pegs"() -> (w448:dbl)
              n134 = And(x=w481, y=w479) -> (x .and. y?=w480:bool)
              n135 = control-ref of="Hopper  Actuator"() -> (w501:refnum<vi>)
              n136 = control-ref of="Reject Solenoid"() -> (w500:refnum<vi>)
              n137 = control-ref of="Sort Solenoid"() -> (w502:refnum<vi>)
              n138 = control-ref of="Feeder Light"() -> (w503:refnum<vi>)
              n139 = control-ref of="Belt Light"() -> (w504:refnum<vi>)
              n140 = case shown="True" w480 {
                frame False {
                }
                frame True {
                  n141 = local write "Program Control"(TRUE) -> ()
                }
              }
              n142 = control-ref of="Pegs Left"() -> (w466:refnum<vi>)
              n143 = control-ref of="Rings Left"() -> (w465:refnum<vi>)
              n144 = call "RejectionArea.vi"("No. Success"=w473, "No. Peg Rej"=w471, "Pegs"=w463, "Current Rej Area Data"=w469, "No. Ring Rej"=w474, "Pegs Left"=w466, "Rej Cntrl"=w470, "Rings Left"=w465, "Program Control"=w472, "No. Failed"=w475, "Rings"=w464, "Prev Rej Area Data"=w468) -> ("Rejector Output"=w467:bool)  [unwired: 3 in]
              n145 = Subtract(x=w448, y=w451) -> (x-y=w450:dbl)
              n146 = Subtract(x=w447, y=w452) -> (x-y=w449:dbl)
              n147 = local write "Pegs Left"(w450) -> ()
              n148 = local write "Rings Left"(w449) -> ()
              n149 = call "ActuatorControls.vi"("Boolean in"=w504, "reference in"=w503, "Sort  Control"="Sort  Control", "Reject Control"="Reject Control", "reference 3"=w502, "reference 4"=w501, "reference 5"=w500, "Feeder Control"="Feeder Control", "Belt Control"="Belt Control", "Hopper Control"="Hopper Control") -> ("Feeder Light"=w526:bool, "Reject Solenoid"=w508:bool, "Belt Light"=w527:bool, "Sort Solenoid"=w507:bool, "Hopper  Actuator"=w506:bool)  [unwired: 1 in]
              n150 = Or(x=w505, y=w507) -> (x .or. y?=w497:bool)
              n151 = Or(x=w467, y=w508) -> (x .or. y?=w498:bool)
              n152 = Or(x=w442, y=w506) -> (x .or. y?=w499:bool)
              n153 = local write "Sort Solenoid"(w497) -> ()
              n154 = local write "Reject Solenoid"(w498) -> ()
              n155 = local write "Hopper  Actuator"(w499) -> ()
            }
            frame "Pause" {
              w533 = FALSE  # Belt Control
              w535 = FALSE  # Feeder Control
              # "Pause Routine:  This routine saves the program variables and goes into a semi-idle mode"
              n156 = Wait (ms)(milliseconds to wait=u32 200 ("millisecond timer value")) -> ()  [unwired: 1 out]
              n157 = local write "Feeder Light"(w533) -> ()
              n158 = local write "Belt Light"(w535) -> ()
              n159 = local read "Feeder Light"() -> (w532:bool)
              n160 = local read "Belt Light"() -> (w534:bool)
            }
            frame "Stop" {
              w538 = TRUE  # Stop Program
              # "Stop Routine: This routine stops and resets all the data collected. It also generates the results of the run"
              n161 = Wait (ms)(milliseconds to wait=u32 50 ("millisecond timer value")) -> ()  [unwired: 1 out]
            }
            frame "Stop Program" {
              w542 = TRUE  # Stop
              w541 = TRUE  # ABORT
              # "Abort Program Routine: This will instantly shut down the program"
            }
          }
          n162 = call-poly <vilib>:"DAQmx Read.vi"("task/channels in"=w392, "error in"=w405) -> ("task out"=w404:refnum<k21>, "data"=w334:bool, "error out"=w402:errorcluster)  [unwired: 11 in]
        }
        event "On light", "Play Button": Value Change {
          w548 = FALSE ("Pause light")
          # "Set the UI elements for the Play state"
          n163 = event-data() -> ()  [unwired: 1 in, 1 out]
          n164 = local write "On light"(TRUE ("On light")) -> ()
          n165 = Wait (ms)(milliseconds to wait=u32 200 ("millisecond timer value")) -> ()  [unwired: 1 out]
          n166 = local write "Pause light"(w548) -> ()
          n167 = local write "Off Light"(w548) -> ()
          n168 = property on="Stop Button" class="Bool"("DisabledEnum"=T2."Enabled" ("Disabled")) -> ()  [unwired: 2 in, 2 out]
          n169 = property on="Reset Button" class="Bool"("DisabledEnum"=T2."Enabled" ("Disabled")) -> ()  [unwired: 2 in, 2 out]
          n170 = property on="Pause Button" class="Bool"("DisabledEnum"=T2."Enabled" ("Disabled")) -> ()  [unwired: 2 in, 2 out]
          n171 = property on="Play Button" class="Bool"("DisabledEnum"=T2."Disabled and Grayed Out" ("Disabled")) -> ()  [unwired: 2 in, 2 out]
        }
        event "Stop Button", "Off Light": Value Change {
          w556 = FALSE ("On light")
          # "Set the UI elements for the Stop state"
          n172 = event-data() -> ()  [unwired: 1 in, 1 out]
          n173 = local write "Off Light"(TRUE ("Off Light")) -> ()
          n174 = Wait (ms)(milliseconds to wait=u32 200 ("millisecond timer value")) -> ()  [unwired: 1 out]
          n175 = local write "Pause light"(w556) -> ()
          n176 = local write "On light"(w556) -> ()
          n177 = property on="Play Button" class="Bool"("DisabledEnum"=T2."Enabled" ("Disabled")) -> ()  [unwired: 2 in, 2 out]
          n178 = property on="Reset Button" class="Bool"("DisabledEnum"=T2."Disabled and Grayed Out" ("Disabled")) -> ()  [unwired: 2 in, 2 out]
          n179 = property on="Stop Button" class="Bool"("DisabledEnum"=T2."Disabled and Grayed Out" ("Disabled")) -> ()  [unwired: 2 in, 2 out]
          n180 = property on="Pause Button" class="Bool"("DisabledEnum"=T2."Disabled and Grayed Out" ("Disabled")) -> ()  [unwired: 2 in, 2 out]
        }
        event "Pause Button": Value Change {
          w564 = FALSE ("On light")
          # "Set the UI elements for the Pause start"
          n181 = event-data() -> ()  [unwired: 1 in, 1 out]
          n182 = local write "Pause light"(TRUE ("Pause light")) -> ()
          n183 = Wait (ms)(milliseconds to wait=u32 200 ("millisecond timer value")) -> ()  [unwired: 1 out]
          n184 = local write "On light"(w564) -> ()
          n185 = local write "Program Control"(w564) -> ()
          n186 = local write "Off Light"(w564) -> ()
          n187 = property on="Stop Button" class="Bool"("DisabledEnum"=T2."Enabled" ("Disabled")) -> ()  [unwired: 2 in, 2 out]
          n188 = property on="Reset Button" class="Bool"("DisabledEnum"=T2."Enabled" ("Disabled")) -> ()  [unwired: 2 in, 2 out]
          n189 = property on="Play Button" class="Bool"("DisabledEnum"=T2."Enabled" ("Disabled")) -> ()  [unwired: 2 in, 2 out]
          n190 = property on="Pause Button" class="Bool"("DisabledEnum"=T2."Disabled and Grayed Out" ("Disabled")) -> ()  [unwired: 2 in, 2 out]
        }
        event "Abort & Exit Button": Value Change {
          w572 = FALSE ("On light")
          # "Set the UI elements for the Stop state"
          n191 = event-data() -> ()  [unwired: 1 in, 1 out]
          n192 = local write "Off Light"(TRUE ("Off Light")) -> ()
          n193 = Wait (ms)(milliseconds to wait=u32 200 ("millisecond timer value")) -> ()  [unwired: 1 out]
          n194 = local write "On light"(w572) -> ()
          n195 = local write "Pause light"(w572) -> ()
          n196 = property on="Play Button" class="Bool"("DisabledEnum"=T2."Enabled" ("Disabled")) -> ()  [unwired: 2 in, 2 out]
          n197 = property on="Stop Button" class="Bool"("DisabledEnum"=T2."Disabled and Grayed Out" ("Disabled")) -> ()  [unwired: 2 in, 2 out]
          n198 = property on="Pause Button" class="Bool"("DisabledEnum"=T2."Disabled and Grayed Out" ("Disabled")) -> ()  [unwired: 2 in, 2 out]
          n199 = property on="Reset Button" class="Bool"("DisabledEnum"=T2."Disabled and Grayed Out" ("Disabled")) -> ()  [unwired: 2 in, 2 out]
        }
        event "Reset Button": Value Change {
          w577 = FALSE ("Peg Flag")
          w582 = 0.0 ("Hopper Status")
          # "Reset all data values of the program"
          n200 = event-data() -> ()  [unwired: 1 in, 1 out]
          n201 = local write "Rejection Control"(i8 0 ("Rejection Control")) -> ()
          n202 = Wait (ms)(milliseconds to wait=u32 200 ("millisecond timer value")) -> ()  [unwired: 1 out]
          n203 = local write "Assembly Flag"(w577) -> ()
          n204 = local write "Peg Flag"(w577) -> ()
          n205 = local write "Program Control"(w577) -> ()
          n206 = local write "Rings"(w582) -> ()
          n207 = local write "Pegs"(w582) -> ()
          n208 = local write "No. Rejected"(w582) -> ()
          n209 = local write "No.  Assembled"(w582) -> ()
          n210 = local write "No. Pegs Rej"(w582) -> ()
          n211 = local write "No. Rings Rej"(w582) -> ()
          n212 = local write "Ring Queue"(w582) -> ()
          n213 = property on="Reset Button" class="Bool"("DisabledEnum"=T2."Enabled" ("Disabled")) -> ()  [unwired: 2 in, 2 out]
          n214 = property on="Pause Button" class="Bool"("DisabledEnum"=T2."Enabled" ("Disabled")) -> ()  [unwired: 2 in, 2 out]
          n215 = property on="Stop Button" class="Bool"("DisabledEnum"=T2."Enabled" ("Disabled")) -> ()  [unwired: 2 in, 2 out]
          n216 = property on="Play Button" class="Bool"("DisabledEnum"=T2."Disabled and Grayed Out" ("Disabled")) -> ()  [unwired: 2 in, 2 out]
        }
      }
      "State" <- w214
    }
  }
  n217 = call <vilib>:"DAQmx Stop Task.vi"("task/channels in"=w102, "error in"=w127) -> ("task out"=w140:refnum<k21>, "error out"=w139:errorcluster)  [unwired: 12 in]
  n218 = call <vilib>:"DAQmx Stop Task.vi"("task/channels in"=w5, "error in"=w4) -> ("task out"=w27:refnum<k21>, "error out"=w26:errorcluster)  [unwired: 12 in]
  n219 = call <vilib>:"DAQmx Stop Task.vi"("task/channels in"=w13, "error in"=w12) -> ("task out"=w34:refnum<k21>, "error out"=w35:errorcluster)  [unwired: 12 in]
  n220 = call <vilib>:"DAQmx Stop Task.vi"("task/channels in"=w7, "error in"=w6) -> ("task out"=w29:refnum<k21>, "error out"=w28:errorcluster)  [unwired: 12 in]
  n221 = call <vilib>:"DAQmx Stop Task.vi"("task/channels in"=w103, "error in"=w117) -> ("task out"=w144:refnum<k21>, "error out"=w143:errorcluster)  [unwired: 12 in]
  n222 = call <vilib>:"DAQmx Stop Task.vi"("task/channels in"=w15, "error in"=w14) -> ("task out"=w36:refnum<k21>, "error out"=w37:errorcluster)  [unwired: 12 in]
  n223 = call <vilib>:"DAQmx Stop Task.vi"("task/channels in"=w119, "error in"=w120) -> ("task out"=w132:refnum<k21>, "error out"=w131:errorcluster)  [unwired: 12 in]
  n224 = call <vilib>:"DAQmx Stop Task.vi"("task/channels in"=w124, "error in"=w123) -> ("task out"=w136:refnum<k21>, "error out"=w135:errorcluster)  [unwired: 12 in]
  n225 = call <vilib>:"DAQmx Stop Task.vi"("task/channels in"=w23, "error in"=w22) -> ("task out"=w45:refnum<k21>, "error out"=w44:errorcluster)  [unwired: 12 in]
  n226 = call <vilib>:"DAQmx Stop Task.vi"("task/channels in"=w21, "error in"=w20) -> ("task out"=w42:refnum<k21>, "error out"=w43:errorcluster)  [unwired: 12 in]
  n227 = call <vilib>:"DAQmx Stop Task.vi"("task/channels in"=w17, "error in"=w16) -> ("task out"=w38:refnum<k21>, "error out"=w39:errorcluster)  [unwired: 12 in]
  n228 = call <vilib>:"DAQmx Stop Task.vi"("task/channels in"=w19, "error in"=w18) -> ("task out"=w40:refnum<k21>, "error out"=w41:errorcluster)  [unwired: 12 in]
  n229 = call <vilib>:"DAQmx Stop Task.vi"("task/channels in"=w47, "error in"=w46) -> ("task out"=w107:refnum<k21>, "error out"=w106:errorcluster)  [unwired: 12 in]
  n230 = call <vilib>:"DAQmx Stop Task.vi"("task/channels in"=w9, "error in"=w8) -> ("task out"=w31:refnum<k21>, "error out"=w30:errorcluster)  [unwired: 12 in]
  n231 = call <vilib>:"DAQmx Stop Task.vi"("task/channels in"=w11, "error in"=w10) -> ("task out"=w32:refnum<k21>, "error out"=w33:errorcluster)  [unwired: 12 in]
  n232 = call <vilib>:"DAQmx Stop Task.vi"("task/channels in"=w3, "error in"=w2) -> ("task out"=w25:refnum<k21>, "error out"=w24:errorcluster)  [unwired: 12 in]
  n233 = call <vilib>:"DAQmx Clear Task.vi"("task in"=w140, "error in"=w139) -> ()  [unwired: 13 in, 1 out]
  n234 = call <vilib>:"DAQmx Clear Task.vi"("task in"=w27, "error in"=w26) -> ()  [unwired: 13 in, 1 out]
  n235 = call <vilib>:"DAQmx Clear Task.vi"("task in"=w34, "error in"=w35) -> ()  [unwired: 13 in, 1 out]
  n236 = call <vilib>:"DAQmx Clear Task.vi"("task in"=w29, "error in"=w28) -> ()  [unwired: 13 in, 1 out]
  n237 = call <vilib>:"DAQmx Clear Task.vi"("task in"=w144, "error in"=w143) -> ()  [unwired: 13 in, 1 out]
  n238 = call <vilib>:"DAQmx Clear Task.vi"("task in"=w36, "error in"=w37) -> ()  [unwired: 13 in, 1 out]
  n239 = call <vilib>:"DAQmx Clear Task.vi"("task in"=w132, "error in"=w131) -> ()  [unwired: 13 in, 1 out]
  n240 = call <vilib>:"DAQmx Clear Task.vi"("task in"=w136, "error in"=w135) -> ()  [unwired: 13 in, 1 out]
  n241 = call <vilib>:"DAQmx Clear Task.vi"("task in"=w45, "error in"=w44) -> ()  [unwired: 13 in, 1 out]
  n242 = call <vilib>:"DAQmx Clear Task.vi"("task in"=w42, "error in"=w43) -> ()  [unwired: 13 in, 1 out]
  n243 = call <vilib>:"DAQmx Clear Task.vi"("task in"=w38, "error in"=w39) -> ()  [unwired: 13 in, 1 out]
  n244 = call <vilib>:"DAQmx Clear Task.vi"("task in"=w40, "error in"=w41) -> ()  [unwired: 13 in, 1 out]
  n245 = call <vilib>:"DAQmx Clear Task.vi"("task in"=w107, "error in"=w106) -> ()  [unwired: 13 in, 1 out]
  n246 = call <vilib>:"DAQmx Clear Task.vi"("task in"=w31, "error in"=w30) -> ()  [unwired: 13 in, 1 out]
  n247 = call <vilib>:"DAQmx Clear Task.vi"("task in"=w32, "error in"=w33) -> ()  [unwired: 13 in, 1 out]
  n248 = call <vilib>:"DAQmx Clear Task.vi"("task in"=w25, "error in"=w24) -> ()  [unwired: 13 in, 1 out]
